vi "GOMDBTS2048 calib Wavelength Calculate Mapping.vi"(8 "error in (no error)":errorcluster, 11 "handle":i32) -> (0 "error out":errorcluster, 2 "function return":i32, 3 "mapping":dbl[](array[numeric]))   [LabVIEW 2015, in "GOMDBTS2048.lvlib"]
doc: "GOBTS2048DLL int __stdcall GOMDBTS2048_calibGetFilterAssignment(int handle, int* value);"
uses:
  GOMDBTS2048.lvlib
  runtime/GOMDBTS2048.dll
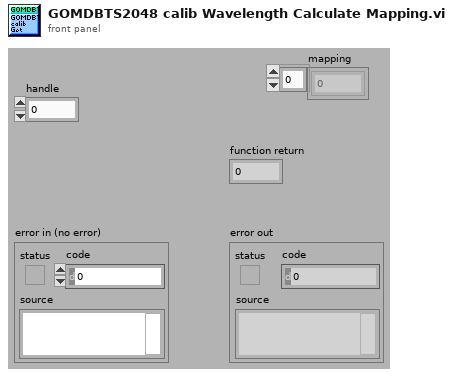
[diagram p1: front panel]
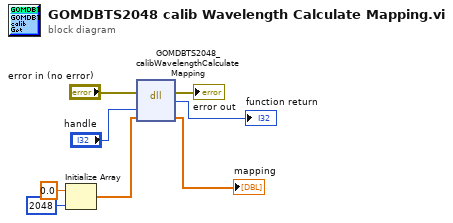
[diagram p0: block diagram]
diagram:
  n1 = Initialize Array(0.0 ("element"), 2048 ("dimension size")) -> (w2:dbl[])
  n2 = dll-call lib="C:/Users/rkoch/Documents/GO_Library/runtime/GOMDBTS2048.*" fn="GOMDBTS2048_calibWavelengthCalculateMapping"(error in="error in (no error)", "handle"="handle", "mapping"=w2) -> (error out=→"error out":errorcluster, "return type"=→"function return":i32, "mapping"=→"mapping":dbl[])  [unwired: 3 in, 1 out]
